vi "Read Child Actor Attributes.vi"(7 "Actor in":refnum<class "Actor.lvclass">) -> (2 "Child Actor Attributes":refnum<data-value>)   [LabVIEW 2020, in "jettl.lvlib"]
uses:
  jettl.lvlib
  Msg/Msg.lvclass
  Actor/Actor.lvclass
  Refs/Refs.lvclass
  Msg Input/Msg Input.lvclass
  Msg Output/Msg Output.lvclass
  Msg Set.ctl
  Unified Actor.ctl
  Child Unified Actor.ctl
  Unified Actor Relation.ctl
  Teller.ctl
  Msg.ctl
  Msgs.ctl
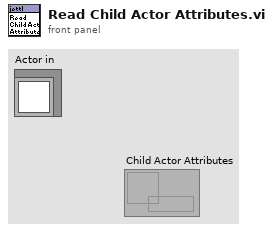
[diagram p1: front panel]
types:
  T1 = typedef "jettl.lvlib/Child Unified Actor.ctl" = map{string, T2}
  T2 = typedef "jettl.lvlib/Unified Actor.ctl" = cluster{"Msgs":T3, "Leaf":bool, "Edge Actors":refnum<class "Actor.lvclass">[], "Core Actors":refnum<class "Actor.lvclass">[], "Root":bool, "Alias":string, "UID":i32, "Transport":refnum<user-event>, "Address":refnum<event-registration>, "This VI":refnum<vi>}
  T3 = typedef "jettl.lvlib/Msgs.ctl" = cluster{"Inbound":T4, "Outbound":T4, "Implemented":T4, "Tell Init":T4, "Tell Init Self":T4, "Tell Init Parent":T4, "Tell Init Child":T4, "Tell Forward":T4, "Tell Forward Self":T4, "Tell Forward Parent":T4, "Tell Forward Child":T4}
  T4 = typedef "jettl.lvlib/Msg Set.ctl" = set{refnum<class "Msg.lvclass">}
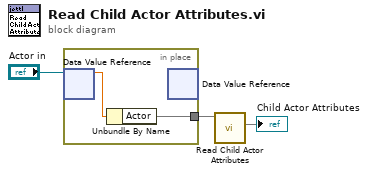
[diagram p0: block diagram]
diagram:
  n1 = in-place {
    in-place-border: [w4] -> w1
    n2 = in-place-dvr #1("Actor in") -> (w5:dbl)  [unwired: 1 out]
    n3 = Unbundle By Name(w5) -> ("Actor"=w4)
    n4 = in-place-dvr #1() -> ()  [unwired: 1 in, 2 out]
  }
  n5 = call-dynamic "Read Child Actor Attributes.vi"("Actor in"=w1) -> ("Child Actor Attributes"=→"Child Actor Attributes":T1)  [unwired: 10 in]
